vi "Counter Setup Freq Mode.vi"(8 "error in":errorcluster, 10 "setup":T1={"Coupling (0:AC)"=enum."DC", "Trigger Slope (0:Positive)"=enum."Negative", "Sensitivity (0:High)"=enum."Medium", "Trigger level [%]"=0.0, "Filter"=FALSE, "Attenuate"=FALSE, "Integration [s]"=1.0, "Ext clock"=FALSE}, 11 "counter session in":T5) -> (0 "error out":errorcluster, 3 "counter session out":T5)   [LabVIEW 2018, in "Counter.lvlib"]
doc: "Call this to initialize counter to frequency measurement."
uses:
  Counter.lvlib
  Counter Session.ctl
  Counter Type.ctl
  Counter Freq Mode Setup.ctl
  Counter Coupling Mode.ctl
  Counter Trigger Edge.ctl
  Counter Sensitivity.ctl
  Picotest U62XXA/PICOTEST U62XXA series.lvlib
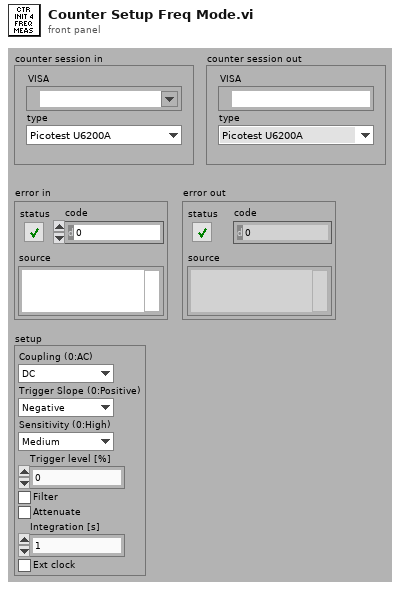
[diagram p1: front panel]
types:
  T1 = typedef "Counter.lvlib/Counter Freq Mode Setup.ctl" = cluster{"Coupling (0:AC)":T2, "Trigger Slope (0:Positive)":T3, "Sensitivity (0:High)":T4, "Trigger level [%]":dbl, "Filter":bool, "Attenuate":bool, "Integration [s]":dbl, "Ext clock":bool}
  T2 = typedef "Counter.lvlib/Counter Coupling Mode.ctl" = enum16{"AC", "DC"}
  T3 = typedef "Counter.lvlib/Counter Trigger Edge.ctl" = enum16{"Positive", "Negative"}
  T4 = typedef "Counter.lvlib/Counter Sensitivity.ctl" = enum16{"High", "Medium", "Low"}
  T5 = typedef "Counter.lvlib/Counter Session.ctl" = cluster{"VISA":refnum<visa-resource-name>, "type":T6}
  T6 = typedef "Counter.lvlib/Counter Type.ctl" = enum16{"Picotest U6200A", "dummy"}
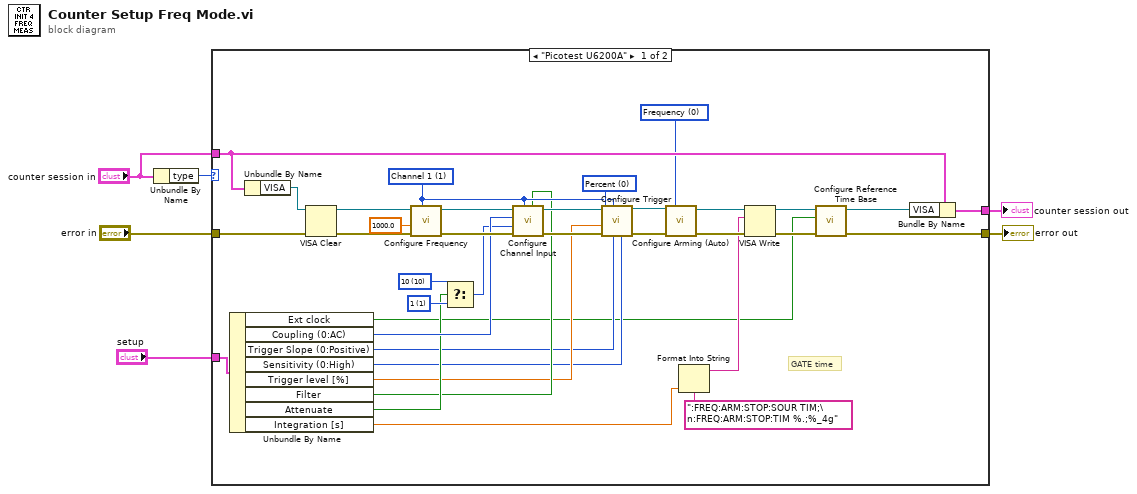
[diagram p0: block diagram]
diagram:
  n1 = Unbundle By Name("counter session in") -> ("type"=w6:T6)
  n2 = case shown="\"Picotest U6200A\"" w6 {
    tunnel: "error in" -> [w40 w44]
    tunnel: "counter session in" -> [w42 w43]
    tunnel: [w8 w44] -> w4
    tunnel: [w41 w43] -> w2
    tunnel: "setup" -> [w30 _]
    frame "Picotest U6200A" {
      w18 = 0 items=["Frequency", "Frequency Ratio", "Period", "Totalize", "Phase", "Edge Rise Time", "Edge Fall Time", "Positive Pulse Width", "Negative Pulse Width", "Duty Cycle", "Time Interval", "Volt Maximum", "Volt Minimum"] ("Measurement (0:Frequency)")
      w27 = u16 10 items=["1"=1, "10"=10] ("Attenuation (1)")
      w28 = u16 1 items=["1"=1, "10"=10] ("Attenuation (1)")
      w32 = 0 items=["Percent", "Volts"] ("Trigger Level Type (0:Percent)")
      w31 = 1 items=["Channel 1"=1, "Channel 2"=2, "Channel 3"=3] ("Channel (1:Channel 1)")
      # "GATE time"
      n3 = Unbundle By Name(w30) -> ("Ext clock"=w7:bool, "Coupling (0:AC)"=w29:T2, "Trigger Slope (0:Positive)"=w22:T3, "Sensitivity (0:High)"=w21:T4, "Trigger level [%]"=w23:dbl, "Filter"=w24:bool, "Attenuate"=w26:bool, "Integration [s]"=w12:dbl)
      n4 = Unbundle By Name(w42) -> ("VISA"=w39:refnum<visa-resource-name>)
      n5 = VISA Clear(VISA resource name=w39, error in (no error)=w40) -> (VISA resource name out=w37:refnum<visa-resource-name>, error out=w38:errorcluster)
      n6 = call "Configure Frequency.vi"("Channel (1:Channel 1)"=w31, "error in (no error)"=w38, "Frequency Estimate (10E+6 Hz)"=1000.0, "VISA resource name"=w37) -> ("error out"=w36:errorcluster, "VISA resource name out"=w35:refnum<visa-resource-name>)  [unwired: 6 in]
      n7 = Select(t=w27, s=w26, f=w28) -> (s? t:f=w25:u16)
      n8 = call "Configure Channel Input.vi"("Enable Filter (Disable)"=w24, "Channel (1:Channel 1)"=w31, "error in (no error)"=w36, "Attenuation (1)"=w25, "Coupling (0:AC)"=w29, "VISA resource name"=w35) -> ("error out"=w34:errorcluster, "VISA resource name out"=w33:refnum<visa-resource-name>)  [unwired: 4 in]
      n9 = call "Configure Trigger.vi"("Sensitivity (0:High)"=w21, "Trigger Slope (0:Positive)"=w22, "Channel (1:Channel 1)"=w31, "error in (no error)"=w34, "Trigger Level (50%)"=w23, "Trigger Level Type (0:Percent)"=w32, "VISA resource name"=w33) -> ("error out"=w20:errorcluster, "VISA resource name out"=w19:refnum<visa-resource-name>)  [unwired: 3 in]
      n10 = call "Configure Arming (Auto).vi"("VISA resource name"=w19, "Measurement (0:Frequency)"=w18, "error in (no error)"=w20) -> ("VISA resource name out"=w15:refnum<visa-resource-name>, "error out"=w16:errorcluster)  [unwired: 11 in]
      n11 = Format Into String(format string=":FREQ:ARM:STOP:SOUR TIM;\n:FREQ:ARM:STOP:TIM %.;%_4g", w12) -> (resulting string=w13:string)  [unwired: 2 in, 1 out]
      n12 = VISA Write(VISA resource name=w15, write buffer=w13, error in (no error)=w16) -> (VISA resource name out=w10:refnum<visa-resource-name>, error out=w11:errorcluster)  [unwired: 1 out]
      n13 = call "Configure Reference Time Base.vi"("error in (no error)"=w11, "External ref. enable (True)"=w7, "VISA resource name"=w10) -> ("error out"=w8:errorcluster, "VISA resource name out"=w9:refnum<visa-resource-name>)  [unwired: 7 in]
      n14 = Bundle By Name(cluster=w42, "VISA"=w9) -> (w41:T5)
    }
    frame Default {
    }
  }
  "error out" <- w4
  "counter session out" <- w2
